vi "Write and Read Multiple Holding Registers.vi"(4 "read count":u16, 6 "read starting address":u16, 7 "unit ID":u8, 8 "error in":errorcluster, 9 "write values":u16[](array[numeric]), 10 "write starting address":u16, 11 "Modbus instance in":refnum<class "Modbus API.lvclass">) -> (0 "error out":errorcluster, 1 "read values":u16[](array[numeric]), 3 "Modbus instance out":refnum<class "Modbus API.lvclass">)   [LabVIEW 2013, in "Modbus Library - Advance.lvlib" / "Modbus API.lvclass"]
doc: "Writes and reads the values of multiple register values in series. The <b>write values</b> are inserted starting at <b>write starting address</b> and the returned <b>read values</b> consists of <b>read count</b> holding registers starting at <b>read starting address</b>."
uses:
  Modbus API.lvclass
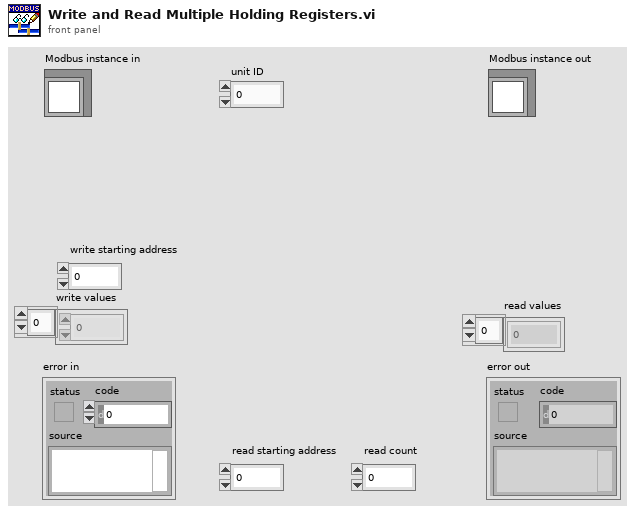
[diagram p1: front panel]
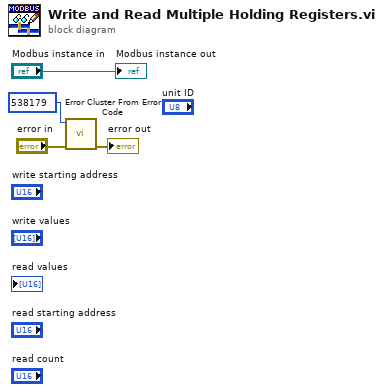
[diagram p0: block diagram]
diagram:
  n1 = call <vilib>:"Error Cluster From Error Code.vi"("error in (no error)"="error in", "error code (0)"=538179) -> ("error out"=→"error out":errorcluster)  [unwired: 7 in]
  "Modbus instance out" <- "Modbus instance in"
